vi "Set Format Into String.vi"(8 "error in (no error)":errorcluster, 9 "# of format strings (0)":i32, 10 "format string":string, 11 "VI in":refnum<vi>) -> (0 "error out":errorcluster, 3 "VI out":refnum<vi>)   [LabVIEW 2016]
uses:
  <vilib>/Utility/traverseref.llb/TRef TravTarget.ctl
  <vilib>/Utility/traverseref.llb/VI Scripting - Traverse.lvlib
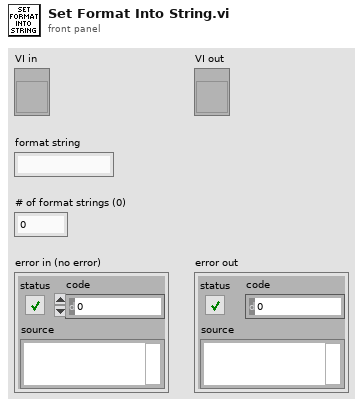
[diagram p1: front panel]
types:
  T1 = typedef "TRef TravTarget.ctl" = enum16{"FP", "BD", "Other"}
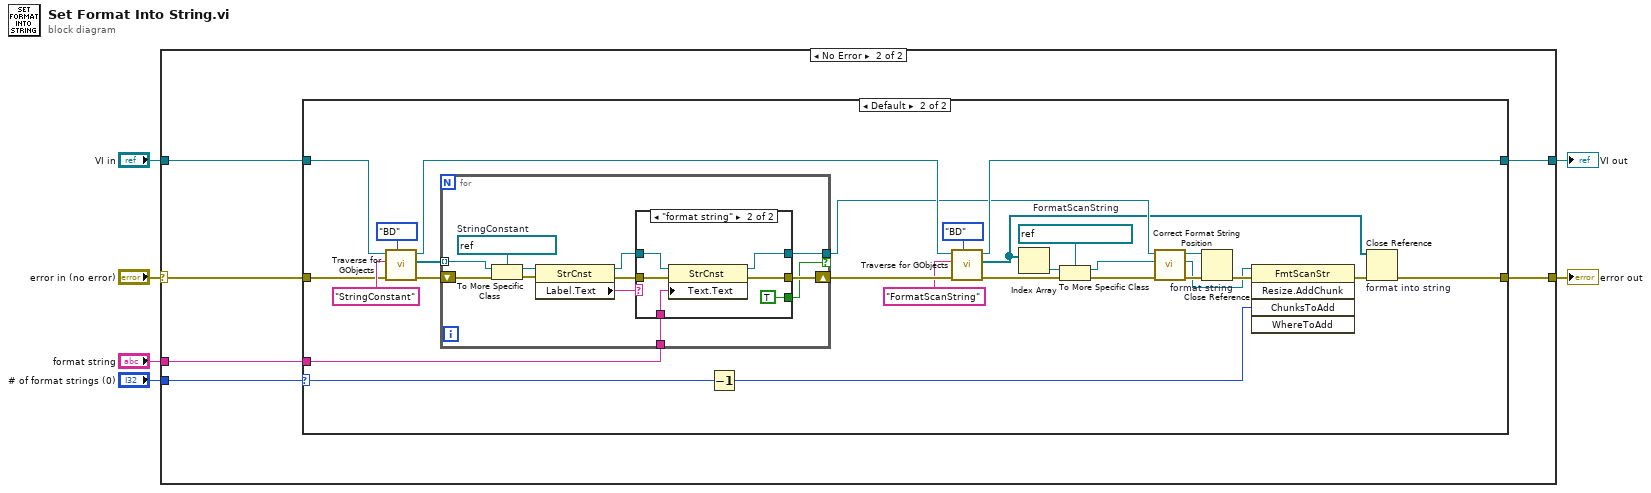
[diagram p0: block diagram]
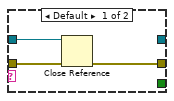
[diagram p4: hidden frame]
diagram:
  n1 = case shown="No Error" "error in (no error)" {
    selector: "error in (no error)" -> [w8 w12]
    tunnel: "VI in" -> [w7 w13]
    tunnel: [w8 w10] -> w4
    tunnel: [w7 w14] -> w3
    tunnel: "format string" -> [_ w11]
    tunnel: "# of format strings (0)" -> [_ w9]
    frame Error {
    }
    frame No Error {
      n2 = case shown="Default" w9 {
        selector: w9 -> [_ w17]
        tunnel: [w16 w42] -> w14
        tunnel: w13 -> [w16 w38]
        tunnel: w12 -> [w15 w34]
        tunnel: w11 -> [_ w33]
        tunnel: [w15 w20] -> w10
        frame ..0 {
        }
        frame Default {
          w32 = refnum<vi> refnum  # FormatScanString
          n3 = call <vilib>:"Traverse for GObjects.vi"("Traverse Target"=TRef_TravTarget."BD", "error in (no error)"=w34, "Class Name"="StringConstant", "VI Refnum"=w38) -> ("error out"=w39:errorcluster, "References"=w36:refnum<vi>[], "dup VI Refnum"=w37:refnum<vi>)  [unwired: 4 in, 1 out]
          n4 = for {
            tunnel: w33 -> [w55]
            tunnel: w36 -> [w48] mode=indexing
            shift-right: [w46] -> w35
            shift-left: w39 -> [w47]
            tunnel: [w45] -> w26 if=w44
            w50 = refnum<vi> refnum  # StringConstant
            n5 = To More Specific Class(target class=w50, reference=w48, error in=w47) -> (specific class reference=w51:refnum<vi>, error out=w52:errorcluster)
            n6 = property class="StrCnst"(reference=w51, error in=w52) -> (reference out=w53:refnum<vi>, error out=w54:errorcluster, "Label.Text"=w49:string)
            n7 = case shown="\"format string\"" w49 {
              tunnel: w54 -> [w58 w64]
              tunnel: w55 -> [_ w63]
              tunnel: w53 -> [w56 w62]
              tunnel: [w57 w61] -> w46
              tunnel: [_ w60] -> w45
              tunnel: [_ TRUE] -> w44
              frame Default {
                n8 = Close Reference(reference=w56, error in (no error)=w58) -> (error out=w57:errorcluster)
              }
              frame "format string" {
                n9 = property class="StrCnst"(reference=w62, error in=w64, "Text.Text"=w63) -> (reference out=w60:refnum<vi>, error out=w61:errorcluster)
              }
            }
          }
          n10 = Decrement(x=w17) -> (x-1=w25:i32)
          n11 = call <vilib>:"Traverse for GObjects.vi"("Traverse Target"=TRef_TravTarget."BD", "error in (no error)"=w35, "Class Name"="FormatScanString", "VI Refnum"=w37) -> ("error out"=w31:errorcluster, "References"=w18:refnum<vi>[], "dup VI Refnum"=w42:refnum<vi>)  [unwired: 4 in, 1 out]
          n12 = Index Array(array=w18) -> (element=w30:refnum<vi>)  [unwired: 1 in]
          n13 = To More Specific Class(target class=w32, reference=w30, error in=w31) -> (specific class reference=w24:refnum<vi>, error out=w23:errorcluster)
          n14 = call "Correct Format String Position.vi"("error in (no error)"=w23, "format into string in"=w24, "format string in"=w26) -> ("error out"=w22:errorcluster, "format into string out"=w21:refnum<vi>, "format string out"=w19:refnum<vi>)  [unwired: 6 in]
          n15 = Close Reference "format string"(reference=w19, error in (no error)=w22) -> (error out=w43:errorcluster)
          n16 = invoke class="FmtScanStr" method="Resize.AddChunk"(reference=w21, error in=w43, "ChunksToAdd"=w25) -> (error out=w27:errorcluster)  [unwired: 2 in, 4 out]
          n17 = Close Reference "format into string"(reference=w18, error in (no error)=w27) -> (error out=w20:errorcluster)
        }
      }
    }
  }
  "error out" <- w4
  "VI out" <- w3
